vi "Stop_acq_and_close_VISA.vi"(2 "error in":errorcluster, 3 "Data flow controls in":T1, 4 "VISA resource name in":refnum<visa-resource-name>) -> (0 "error out":errorcluster, 1 "Data flow controls out":T1)   [LabVIEW 2016]
uses:
  <vilib>/Instr/_visa.llb/VISA Flush IO Buffer Mask.ctl
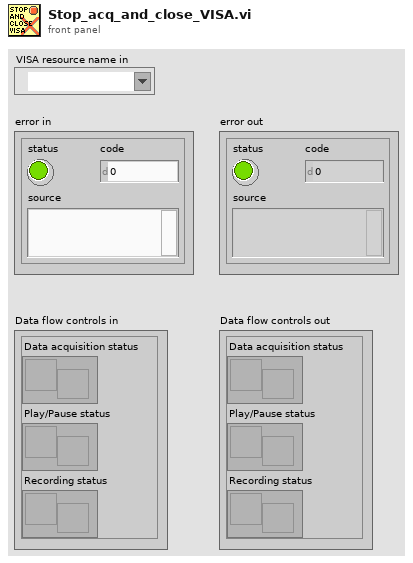
[diagram p1: front panel]
types:
  T1 = cluster{"Data acquisition status":refnum<notifier>, "Play/Pause status":refnum<notifier>, "Recording status":refnum<notifier>}
  T2 = typedef "VISA Flush IO Buffer Mask.ctl" = u16
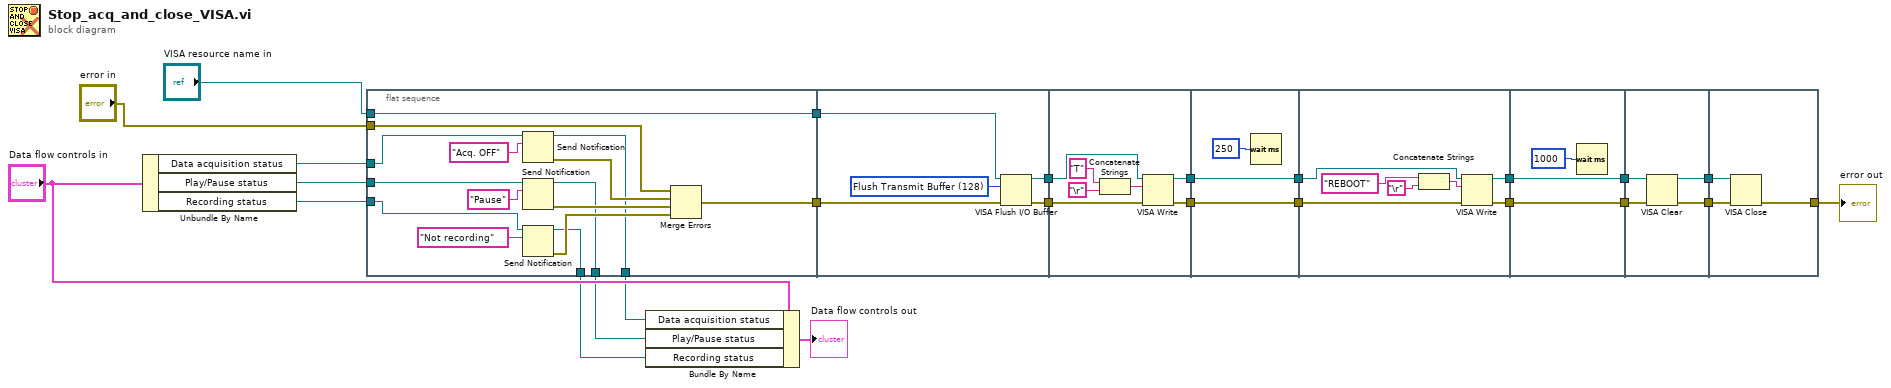
[diagram p0: block diagram]
diagram:
  n1 = Unbundle By Name("Data flow controls in") -> ("Data acquisition status"=w10:refnum<notifier>, "Play/Pause status"=w9:refnum<notifier>, "Recording status"=w8:refnum<notifier>)
  n2 = flat-sequence {
    tunnel: "error in" -> [w37]
    tunnel: "VISA resource name in" -> [w40]
    tunnel: [w40] -> w12
    tunnel: [w36] -> w11
    tunnel: w10 -> [w39]
    tunnel: w9 -> [w38]
    tunnel: w8 -> [w30]
    tunnel: [w28] -> w6
    tunnel: [w27] -> w5
    tunnel: [w26] -> w4
    tunnel: [w42] -> w24
    tunnel: [w41] -> w23
    tunnel: w12 -> [w45]
    tunnel: w11 -> [w43]
    tunnel: w24 -> [w52]
    tunnel: w23 -> [w51]
    tunnel: [w47] -> w21
    tunnel: [w46] -> w19
    tunnel: [w54] -> w22
    tunnel: w21 -> [w54]
    tunnel: [w53] -> w20
    tunnel: w19 -> [w53]
    tunnel: w22 -> [w59]
    tunnel: w20 -> [w58]
    tunnel: [w57] -> w17
    tunnel: [w56] -> w14
    tunnel: [w64] -> w18
    tunnel: w17 -> [w64]
    tunnel: [w63] -> w15
    tunnel: w14 -> [w63]
    tunnel: w18 -> [w69]
    tunnel: [w68] -> w16
    tunnel: w15 -> [w67]
    tunnel: [w66] -> w13
    tunnel: w16 -> [w72]
    tunnel: w13 -> [w71]
    tunnel: [w70] -> w2
    frame #0 {
      n3 = Send Notification(notification="Acq. OFF", notifier=w39) -> (notifier out=w28:refnum<notifier>, error out=w35:errorcluster)  [unwired: 1 in]
      n4 = Send Notification(notification="Pause", notifier=w38) -> (notifier out=w27:refnum<notifier>, error out=w34:errorcluster)  [unwired: 1 in]
      n5 = Send Notification(notification="Not recording", notifier=w30) -> (notifier out=w26:refnum<notifier>, error out=w31:errorcluster)  [unwired: 1 in]
      n6 = Merge Errors(w37, w35, w34, w31) -> (w36:errorcluster)
    }
    frame #1 {
      w44 = T2 128 items=["Flush Receive Buffer"=16, "Write Transmit Buffer to Device"=32, "Flush Receive Buffer (No I/O)"=64, "Flush Transmit Buffer"=128] ("Mask")
      n7 = VISA Flush I/O Buffer(VISA resource name=w45, mask (16)=w44, error in (no error)=w43) -> (VISA resource name out=w42:refnum<visa-resource-name>, error out=w41:errorcluster)
    }
    frame #2 {
      n8 = Concatenate Strings("T" ("write buffer"), "\r") -> (w48:string)
      n9 = VISA Write(VISA resource name=w52, write buffer=w48, error in (no error)=w51) -> (VISA resource name out=w47:refnum<visa-resource-name>, error out=w46:errorcluster)  [unwired: 1 out]
    }
    frame #3 {
      n10 = Wait (ms)(milliseconds to wait=u32 250) -> ()  [unwired: 1 out]
    }
    frame #4 {
      n11 = Concatenate Strings("REBOOT" ("write buffer"), "\r") -> (w60:string)
      n12 = VISA Write(VISA resource name=w59, write buffer=w60, error in (no error)=w58) -> (VISA resource name out=w57:refnum<visa-resource-name>, error out=w56:errorcluster)  [unwired: 1 out]
    }
    frame #5 {
      n13 = Wait (ms)(milliseconds to wait=u32 1000) -> ()  [unwired: 1 out]
    }
    frame #6 {
      n14 = VISA Clear(VISA resource name=w69, error in (no error)=w67) -> (VISA resource name out=w68:refnum<visa-resource-name>, error out=w66:errorcluster)
    }
    frame #7 {
      n15 = VISA Close(VISA resource name=w72, error in (no error)=w71) -> (error out=w70:errorcluster)
    }
  }
  n16 = Bundle By Name(cluster="Data flow controls in", "Data acquisition status"=w6, "Play/Pause status"=w5, "Recording status"=w4) -> (→"Data flow controls out":T1)
  "error out" <- w2
